vi "Array Tests.vi"() -> ()   [LabVIEW 2012]
uses:
  <userlib>/BotSpeak/VIs/Direct/BotSpeak_Control.ctl
  <userlib>/BotSpeak/VIs/Scripting/URAPI_ForStart_num.vi
panel:
  out "response":string="array_SIZE = 10\ncount0 = 0\njunk = 3\narray[count0] = 0\ntest = 3\ncount0 += 1 -> 1\nIf (1 < 9) -> 10\njunk = 3\narray[count0] = 1\ntest = 3\ncount0 += 1 -> 2\nIf (2 < 9) -> 10\njunk = 3\narray[count0] = 2\ntest = 3\ncount0 += 1 -> 3\nIf (3 < 9) -> 10\njunk = 3\narray[count0] = 3\ntest = 3\ncount0 += 1 -> 4\nIf (4 < 9) -> 10\njunk = 3\narray[count0] = 4\ntest = 3\ncount0 += 1 -> 5\nIf (5 < 9) -> 10\njunk = 3\narray[count0] = 5\ntest = 3\ncount0 += 1 -> 6\nIf (6 < 9) -> 10\njunk = 3\narray[count0] = 6\ntest = 3\ncount0 += 1 -> 7\nIf (7 < 9) -> 10\njunk = 3\narray[count0] = 7\ntest = 3\ncount0 += 1 -> 8\nIf (8 < 9) -> 10\njunk = 3\narray[count0] = 8\ntest = 3\ncount0 += 1 -> 9\nIf (9 < 9) -> 10\njunk = 3\narray[count0] = 9\ntest = 3\ncount0 += 1 -> 10\nIf (10 < 9) -> 38\nDone\r"
  out "value 2":string="2\r\n"
  out "variables":string[](array[string])=["VER = 8\r\n", "HI = 1\r\n", "LO = 0\r\n", "test = 3\r\n", "array_SIZE = 10\r\n", "array_0 = 0\r\n", "array_1 = 1\r\n", "array_2 = 2\r\n", "array_3 = 3\r\n", "array_4 = 4\r\n", "array_5 = 5\r\n", "array_6 = 6\r\n", "array_7 = 7\r\n", "array_8 = 8\r\n", "array_9 = 9\r\n", "count0 = 10\r\n", "junk = 3\r\n"]
  out "value":string="2\r\n"
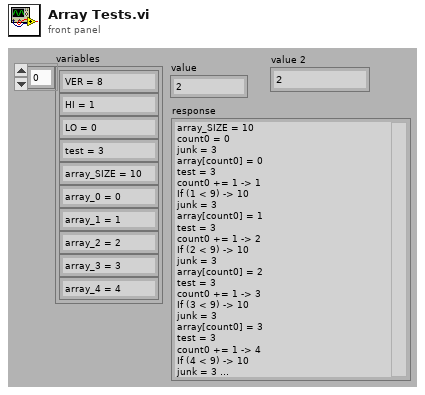
[diagram p1: front panel]
types:
  T1 = typedef "BotSpeak_Control.ctl" = cluster{"Address":string, "Reply EOF":string, "Hardware":path, "Retries":i8, "Timeout":i32}
  T2 = typedef "URAPI_Control.ctl" = cluster{"Script":string, "Whiles":u8[], "Ifs":u8[], "Supress Err":bool, "Errors":string}
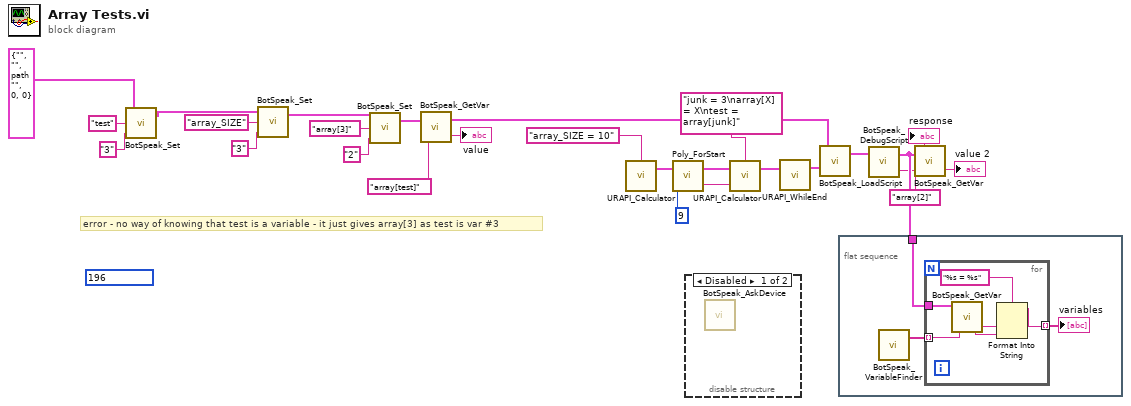
[diagram p0: block diagram]
diagram:
  (unwired) u8 196
  # "error - no way of knowing that test is a variable - it just gives array[3] as test is var #3"
  n1 = call <userlib>:"BotSpeak_Set.vi"("value"="3", "Variable In"="test", "Bot Settings"=T1 {"Address"="", "Reply EOF"="", "Hardware"=path "", "Retries"=0, "Timeout"=0}) -> ("Bot Settings"=w17:T1)  [unwired: 1 out]
  n2 = call <userlib>:"BotSpeak_Set.vi"("value"="3", "Variable In"="array_SIZE", "Bot Settings"=w17) -> ("Bot Settings"=w22:T1)  [unwired: 1 out]
  n3 = call <userlib>:"BotSpeak_Set.vi"("value"="2", "Variable In"="array[3]", "Bot Settings"=w22) -> ("Bot Settings"=w16:T1)  [unwired: 1 out]
  n4 = call <userlib>:"BotSpeak_GetVar.vi"("Variable In"="array[test]", "Bot Settings"=w16) -> ("value"=→"value":string, "Bot Settings out"=w6:T1)
  n5 = call <userlib>:"URAPI_Calculator.vi"("Formula"="array_SIZE = 10") -> ("URAPI Script"=w12:T2)  [unwired: 3 in, 1 out]
  n6 = call-poly <userlib>:"Poly_ForStart.vi"("Iterations"=u8 9, "URAPI Script"=w12) -> ("variable"=w7:string, "URAPI Script Out"=w8:T2)  [unwired: 2 in]
  n7 = disable-structure shown="Disabled" {
    frame Disabled {
      n8 = call <userlib>:"BotSpeak_AskDevice.vi"() -> ()  [unwired: 3 in, 1 out]
    }
    frame Enabled {
    }
  }
  n9 = call <userlib>:"URAPI_Calculator.vi"("X"=w7, "URAPI Script"=w8, "Formula"="junk = 3\narray[X] = X\ntest = array[junk]") -> ("URAPI Script"=w9:T2)  [unwired: 1 in, 1 out]
  n10 = call <userlib>:"URAPI_WhileEnd.vi"("URAPI Script"=w9) -> ("URAPI Script Out"=w10:T2)  [unwired: 4 in]
  n11 = call <userlib>:"BotSpeak_LoadScript.vi"("URAPI Script"=w10, "Bot Settings"=w6) -> ("Bot Settings"=w5:T1)  [unwired: 1 out]
  n12 = flat-sequence {
    tunnel: w2 -> [w29]
    frame #0 {
      n13 = call <userlib>:"BotSpeak_VariableFinder.vi"() -> ("Variables"=w28:string[])  [unwired: 2 in, 1 out]
      n14 = for {
        tunnel: w29 -> [w34]
        tunnel: w28 -> [w31] mode=indexing
        tunnel: [w30] -> w27 mode=indexing
        n15 = call <userlib>:"BotSpeak_GetVar.vi"("Variable In"=w31, "Bot Settings"=w34) -> ("value"=w32:string)  [unwired: 1 out]
        n16 = Format Into String(format string="%s = %s", w31, w32) -> (resulting string=w30:string)  [unwired: 2 in, 1 out]
      }
      "variables" <- w27
    }
  }
  n17 = call <userlib>:"BotSpeak_DebugScript.vi"("Bot Settings"=w5) -> ("response"=→"response":string, "Bot Settings"=w2:T1)  [unwired: 1 in]
  n18 = call <userlib>:"BotSpeak_GetVar.vi"("Variable In"="array[2]", "Bot Settings"=w2) -> ("value"=→"value 2":string)  [unwired: 1 out]
